vi "Timer2.vi"() -> ()   [LabVIEW 2011]
panel:
  out "String":string
  out "path string":string
  out "read text":string
  in  "save":bool
  out "CurrentPath":path=path "C:/Documents and Settings/TGI0362/My Documents/xUserData/LabVIEW_8.x/cmDVT_Factory-BBU-R5"
  in  "stop":bool
  in  "error in":errorcluster
  out "error out 2":errorcluster
  out "VISA resource name out":refnum<visa-resource-name>
  out "error out":errorcluster
  out "VISA resource 2":refnum<visa-resource-name>
  out "P1.0 status(True=ON)":bool
  out "In Range?":bool
  out "hr+min":i32
  out "OFF hr+min":i32
  out "ON hr+min":i32
  out "Today? \n(True=Enable)":bool
  out "week string":string
  out "now week string":string
  out "confilct ? (True=no conflict)":bool
  in  "OFF minute(00-59)":i32
  in  "OFF hour(00-23)":i32
  in  "ON minute(00-59)":i32
  in  "ON hour(00-23)":i32
  in  "Sun":bool
  in  "Sat":bool
  in  "Fri":bool
  in  "Thu":bool
  in  "Wed":bool
  in  "Tue":bool
  in  "Mon":bool
  out "new picture":picture
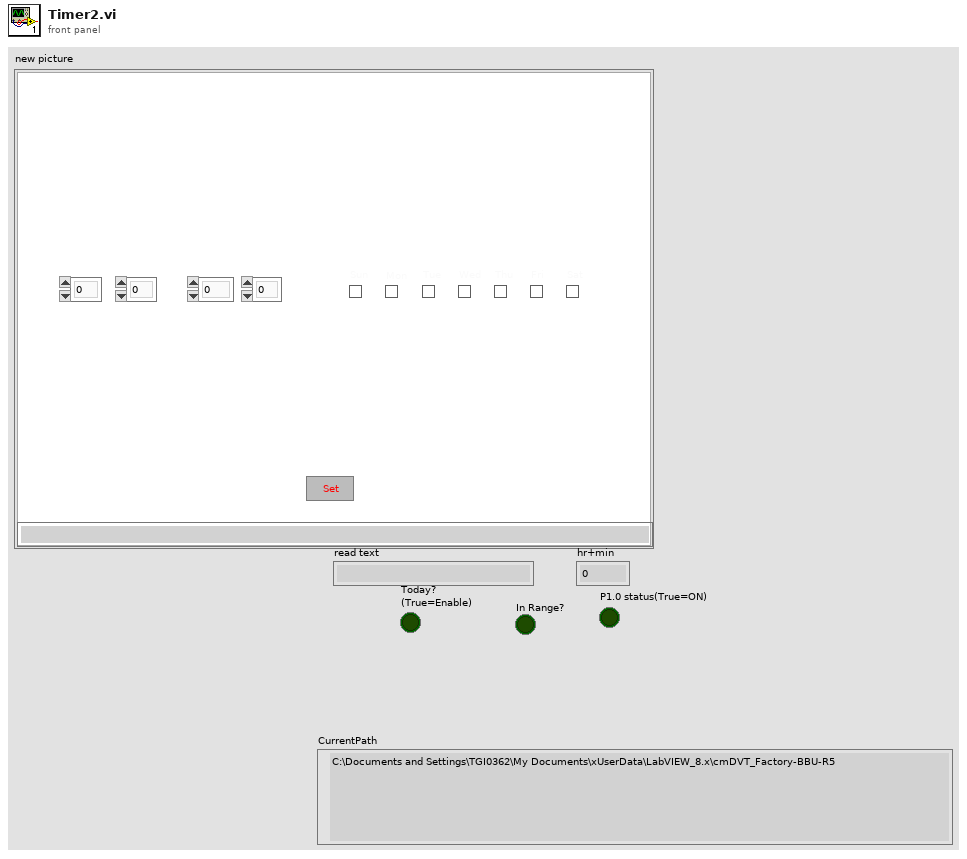
[diagram p1: front panel]
types:
  T1 = typedef "imagedata.ctl" = cluster{"image type":i32, "image depth":i32, "image":u8[], "mask":u8[], "colors":u32[], "Rectangle":cluster{"left":i16, "top":i16, "right":i16, "bottom":i16}}
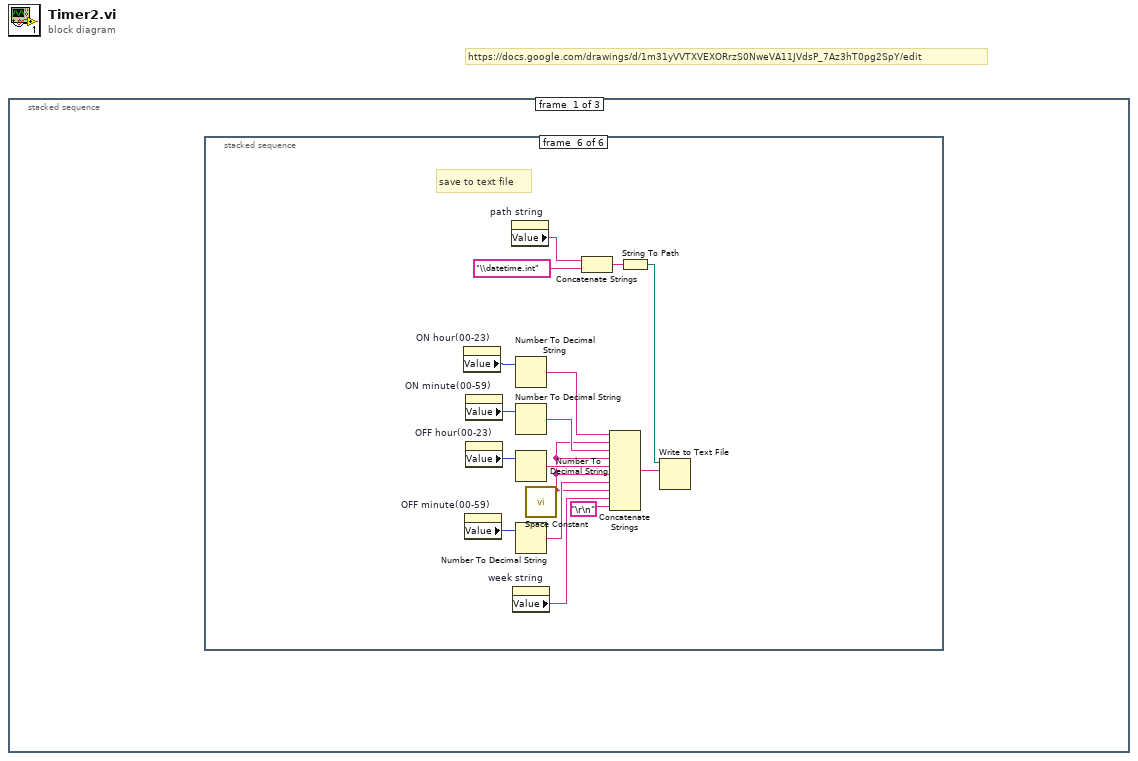
[diagram p0: block diagram]
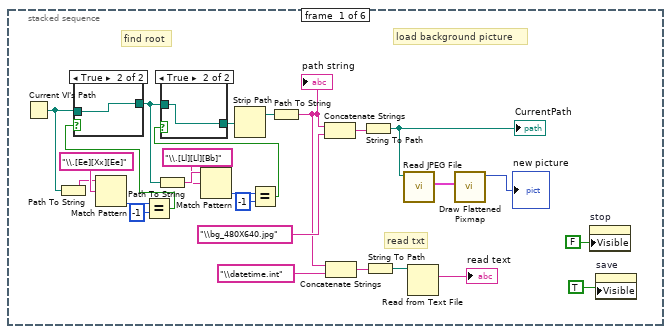
[diagram p2: hidden frame]
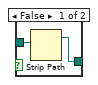
[diagram p3: hidden frame]
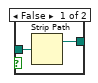
[diagram p4: hidden frame]
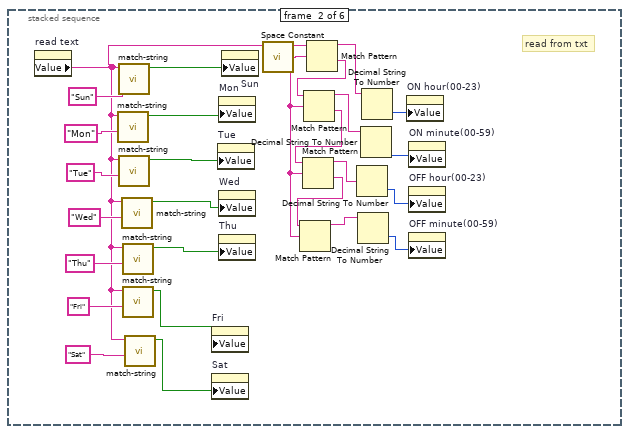
[diagram p5: hidden frame]
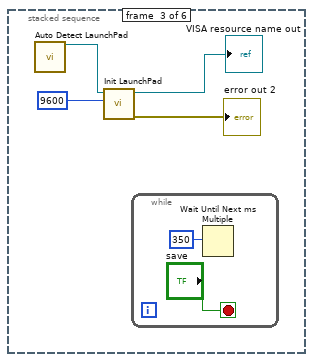
[diagram p6: hidden frame]
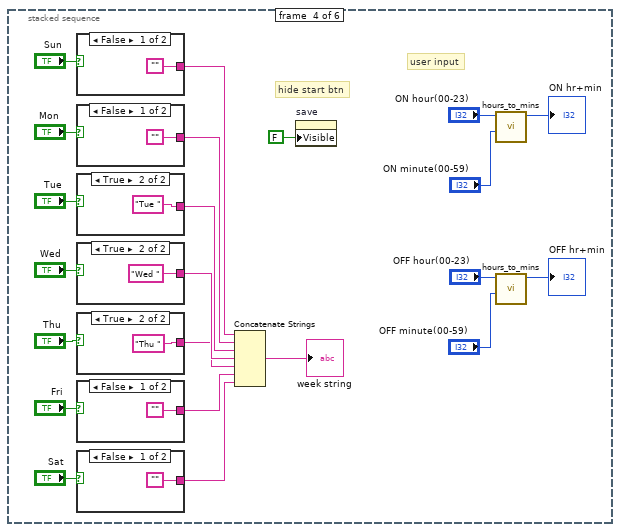
[diagram p7: hidden frame]
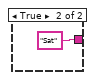
[diagram p8: hidden frame]
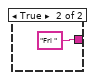
[diagram p9: hidden frame]
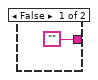
[diagram p10: hidden frame]
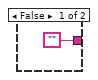
[diagram p11: hidden frame]
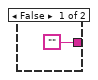
[diagram p12: hidden frame]
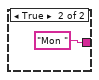
[diagram p13: hidden frame]
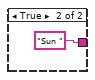
[diagram p14: hidden frame]
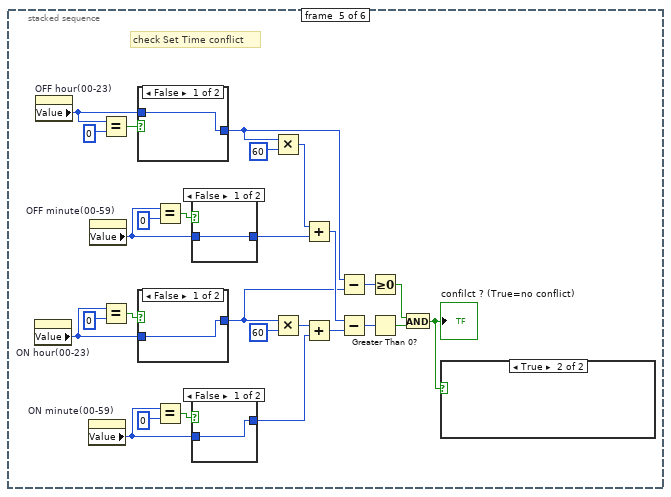
[diagram p15: hidden frame]
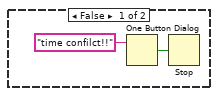
[diagram p16: hidden frame]
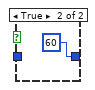
[diagram p17: hidden frame]
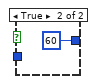
[diagram p18: hidden frame]
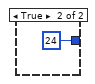
[diagram p19: hidden frame]
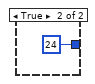
[diagram p20: hidden frame]
diagram:
  # "https://docs.google.com/drawings/d/1m31yVVTXVEXORrzS0NweVA11JVdsP_7Az3hT0pg2SpY/edit"
  n1 = stacked-sequence {
    frame #0 {
      n2 = stacked-sequence {
        frame #0 {
          # "read txt"
          # "load background picture"
          # "find root"
          n3 = Current VI's Path() -> (path=w15:path)
          n4 = Path To String(path=w15) -> (string=w14:string)
          n5 = Match Pattern(string=w14, regular expression="\\.[Ee][Xx][Ee]") -> (offset past match=w12:i32)  [unwired: 1 in, 3 out]
          n6 = Equal?(x=w12, y=-1) -> (x = y?=w24:bool)
          n7 = case shown="True" w24 {
            tunnel: [w30 w32] -> w21
            tunnel: w15 -> [w31 w32]
            frame False {
              n8 = Strip Path(path=w31) -> (stripped path=w30:path)  [unwired: 1 out]
            }
            frame True {
            }
          }
          n9 = Path To String(path=w21) -> (string=w18:string)
          n10 = Match Pattern(string=w18, regular expression="\\.[Ll][Ll][Bb]") -> (offset past match=w20:i32)  [unwired: 1 in, 3 out]
          n11 = Equal?(x=w20, y=-1) -> (x = y?=w23:bool)
          n12 = case shown="True" w23 {
            tunnel: [w27 w29] -> w22
            tunnel: w21 -> [w28 w29]
            frame False {
              n13 = Strip Path(path=w28) -> (stripped path=w27:path)  [unwired: 1 out]
            }
            frame True {
            }
          }
          n14 = Strip Path(path=w22) -> (stripped path=w11:path)  [unwired: 1 out]
          n15 = Path To String(path=w11) -> (string=w1:string)
          "path string" <- w1
          n16 = Concatenate Strings(w1, "\\bg_480X640.jpg") -> (w9:string)
          n17 = Concatenate Strings(w1, "\\datetime.int") -> (w4:string)
          n18 = String To Path(string=w9) -> (path=w8:path)
          "CurrentPath" <- w8
          n19 = String To Path(string=w4) -> (path=w3:path)
          n20 = call <vilib>:"Read JPEG File.vi"("path to JPEG file"=w8) -> ("image data"=w25:T1)  [unwired: 8 in, 2 out]
          n21 = Read from Text File(file (use dialog)=w3) -> (text=→"read text":string)  [unwired: 3 in, 3 out]
          n22 = call <vilib>:"Draw Flattened Pixmap.vi"("image data"=w25) -> ("new picture"=→"new picture":picture)  [unwired: 8 in]
          n23 = property on="stop" class="Bool"("Visible"=FALSE) -> ()  [unwired: 2 in, 2 out]
          n24 = property on="save" class="Bool"("Visible"=TRUE) -> ()  [unwired: 2 in, 2 out]
        }
        frame #1 {
          # "read from txt"
          n25 = property on="read text" class="Str"() -> ("Value"=w45:string)  [unwired: 2 in, 2 out]
          n26 = call "match-string.vi"("match string"="Mon", "String"=w45) -> ("match?(True=match)"=w46:bool)  [unwired: 9 in]
          n27 = call "match-string.vi"("match string"="Sun", "String"=w45) -> ("match?(True=match)"=w59:bool)  [unwired: 9 in]
          n28 = call "match-string.vi"("match string"="Tue", "String"=w45) -> ("match?(True=match)"=w47:bool)  [unwired: 9 in]
          n29 = call "match-string.vi"("match string"="Wed", "String"=w45) -> ("match?(True=match)"=w48:bool)  [unwired: 9 in]
          n30 = call "match-string.vi"("match string"="Thu", "String"=w45) -> ("match?(True=match)"=w49:bool)  [unwired: 9 in]
          n31 = call "match-string.vi"("match string"="Fri", "String"=w45) -> ("match?(True=match)"=w50:bool)  [unwired: 9 in]
          n32 = call "match-string.vi"("match string"="Sat", "String"=w45) -> ("match?(True=match)"=w51:bool)  [unwired: 9 in]
          n33 = property on="Fri" class="Bool (strict)"("Value"=w50) -> ()  [unwired: 2 in, 2 out]
          n34 = property on="Sat" class="Bool (strict)"("Value"=w51) -> ()  [unwired: 2 in, 2 out]
          n35 = property on="Tue" class="Bool (strict)"("Value"=w47) -> ()  [unwired: 2 in, 2 out]
          n36 = property on="Mon" class="Bool (strict)"("Value"=w46) -> ()  [unwired: 2 in, 2 out]
          n37 = property on="Wed" class="Bool (strict)"("Value"=w48) -> ()  [unwired: 2 in, 2 out]
          n38 = property on="Thu" class="Bool (strict)"("Value"=w49) -> ()  [unwired: 2 in, 2 out]
          n39 = property on="Sun" class="Bool (strict)"("Value"=w59) -> ()  [unwired: 2 in, 2 out]
          n40 = call <vilib>:"Space Constant.vi"() -> ("String"=w34:string)
          n41 = Match Pattern(string=w45, regular expression=w34) -> (before substring=w44:string, after substring=w42:string)  [unwired: 1 in, 2 out]
          n42 = Match Pattern(string=w42, regular expression=w34) -> (before substring=w41:string, after substring=w40:string)  [unwired: 1 in, 2 out]
          n43 = Match Pattern(string=w40, regular expression=w34) -> (before substring=w39:string, after substring=w36:string)  [unwired: 1 in, 2 out]
          n44 = Match Pattern(string=w36, regular expression=w34) -> (before substring=w35:string)  [unwired: 1 in, 3 out]
          n45 = Decimal String To Number(string=w39) -> (number=w38:i32)  [unwired: 2 in, 1 out]
          n46 = Decimal String To Number(string=w35) -> (number=w33:i32)  [unwired: 2 in, 1 out]
          n47 = Decimal String To Number(string=w41) -> (number=w37:i32)  [unwired: 2 in, 1 out]
          n48 = Decimal String To Number(string=w44) -> (number=w43:i32)  [unwired: 2 in, 1 out]
          n49 = property on="ON hour(00-23)" class="DigNum (strict)"("Value"=w43) -> ()  [unwired: 2 in, 2 out]
          n50 = property on="ON minute(00-59)" class="DigNum (strict)"("Value"=w37) -> ()  [unwired: 2 in, 2 out]
          n51 = property on="OFF hour(00-23)" class="DigNum (strict)"("Value"=w38) -> ()  [unwired: 2 in, 2 out]
          n52 = property on="OFF minute(00-59)" class="DigNum (strict)"("Value"=w33) -> ()  [unwired: 2 in, 2 out]
        }
        frame #2 {
          n53 = call "Auto Detect LaunchPad.vi"() -> ("VISA resource"=w62:refnum<visa-resource-name>)  [unwired: 14 in, 1 out]
          n54 = call "Init LaunchPad.vi"("Baud Rate (9600)"=u32 9600, "VISA resource"=w62) -> ("error out"=→"error out 2":errorcluster, "VISA resource name out"=→"VISA resource name out":refnum<visa-resource-name>)  [unwired: 8 in]
          n55 = while {
            stop <- "save" stop-if-true
            n56 = Wait Until Next ms Multiple(millisecond multiple=u32 350) -> ()  [unwired: 1 out]
          }
        }
        frame #3 {
          # "hide start btn"
          # "user input"
          n57 = case shown="False" "Sun" {
            tunnel: ["" "Sun "] -> w86
            frame False {
            }
            frame True {
            }
          }
          n58 = case shown="False" "Mon" {
            tunnel: ["" "Mon "] -> w79
            frame False {
            }
            frame True {
            }
          }
          n59 = case shown="True" "Tue" {
            tunnel: ["" "Tue "] -> w78
            frame False {
            }
            frame True {
            }
          }
          n60 = case shown="True" "Wed" {
            tunnel: ["" "Wed "] -> w77
            frame False {
            }
            frame True {
            }
          }
          n61 = case shown="True" "Thu" {
            tunnel: ["" "Thu "] -> w76
            frame False {
            }
            frame True {
            }
          }
          n62 = case shown="False" "Fri" {
            tunnel: ["" "Fri "] -> w75
            frame False {
            }
            frame True {
            }
          }
          n63 = case shown="False" "Sat" {
            tunnel: ["" "Sat"] -> w74
            frame False {
            }
            frame True {
            }
          }
          n64 = Concatenate Strings(w86, w79, w78, w77, w76, w75, w74) -> (→"week string":string)
          n65 = property on="save" class="Bool"("Visible"=FALSE) -> ()  [unwired: 2 in, 2 out]
          n66 = call "hours_to_mins.vi"("minute(00-59)"="ON minute(00-59)", "hour(00-23)"="ON hour(00-23)") -> ("hr+min"=→"ON hr+min":i32)  [unwired: 9 in]
          n67 = call "hours_to_mins.vi"("minute(00-59)"="OFF minute(00-59)", "hour(00-23)"="OFF hour(00-23)") -> ("hr+min"=→"OFF hr+min":i32)  [unwired: 9 in]
        }
        frame #4 {
          # "check Set Time conflict"
          n68 = property on="ON hour(00-23)" class="DigNum (strict)"() -> ("Value"=w121:i32)  [unwired: 2 in, 2 out]
          n69 = property on="OFF hour(00-23)" class="DigNum (strict)"() -> ("Value"=w124:i32)  [unwired: 2 in, 2 out]
          n70 = property on="ON minute(00-59)" class="DigNum (strict)"() -> ("Value"=w118:i32)  [unwired: 2 in, 2 out]
          n71 = property on="OFF minute(00-59)" class="DigNum (strict)"() -> ("Value"=w115:i32)  [unwired: 2 in, 2 out]
          n72 = Equal?(x=w124, y=0) -> (x = y?=w126:bool)
          n73 = Equal?(x=w121, y=0) -> (x = y?=w123:bool)
          n74 = case shown="False" w126 {
            tunnel: [w137 24] -> w111
            tunnel: w124 -> [w137 _]
            frame False {
            }
            frame True {
            }
          }
          n75 = case shown="False" w123 {
            tunnel: [w135 24] -> w105
            tunnel: w121 -> [w135 _]
            frame False {
            }
            frame True {
            }
          }
          n76 = Equal?(x=w115, y=0) -> (x = y?=w117:bool)
          n77 = Equal?(x=w118, y=0) -> (x = y?=w120:bool)
          n78 = case shown="False" w117 {
            tunnel: [w131 60] -> w108
            tunnel: w115 -> [w131 _]
            frame False {
            }
            frame True {
            }
          }
          n79 = case shown="False" w120 {
            tunnel: [w133 60] -> w103
            tunnel: w118 -> [w133 _]
            frame False {
            }
            frame True {
            }
          }
          n80 = Multiply(x=w111, y=60) -> (x*y=w109:i32)
          n81 = Multiply(x=w105, y=60) -> (x*y=w104:i32)
          n82 = Add(x=w109, y=w108) -> (x+y=w107:i32)
          n83 = Add(x=w104, y=w103) -> (x+y=w102:i32)
          n84 = Subtract(x=w111, y=w105) -> (x-y=w128:i32)
          n85 = Subtract(x=w107, y=w102) -> (x-y=w127:i32)
          n86 = Greater Or Equal To 0?(x=w128) -> (x >= 0?=w114:bool)
          n87 = Greater Than 0?(x=w127) -> (x > 0?=w113:bool)
          n88 = And(x=w114, y=w113) -> (x .and. y?=w112:bool)
          "confilct ? (True=no conflict)" <- w112
          n89 = case shown="True" w112 {
            frame False {
              n90 = One Button Dialog(message="time confilct!!") -> (true=w129:bool)  [unwired: 1 in]
              n91 = Stop(stop? (T)=w129) -> ()
            }
            frame True {
            }
          }
        }
        frame #5 {
          # "save to text file"
          n92 = property on="ON hour(00-23)" class="DigNum (strict)"() -> ("Value"=w142:i32)  [unwired: 2 in, 2 out]
          n93 = property on="OFF minute(00-59)" class="DigNum (strict)"() -> ("Value"=w139:i32)  [unwired: 2 in, 2 out]
          n94 = property on="ON minute(00-59)" class="DigNum (strict)"() -> ("Value"=w141:i32)  [unwired: 2 in, 2 out]
          n95 = property on="OFF hour(00-23)" class="DigNum (strict)"() -> ("Value"=w140:i32)  [unwired: 2 in, 2 out]
          n96 = property on="path string" class="Str"() -> ("Value"=w144:string)  [unwired: 2 in, 2 out]
          n97 = property on="week string" class="Str"() -> ("Value"=w150:string)  [unwired: 2 in, 2 out]
          n98 = Number To Decimal String(number=w142) -> (decimal integer string=w154:string)  [unwired: 1 in]
          n99 = Number To Decimal String(number=w141) -> (decimal integer string=w153:string)  [unwired: 1 in]
          n100 = Number To Decimal String(number=w140) -> (decimal integer string=w152:string)  [unwired: 1 in]
          n101 = Number To Decimal String(number=w139) -> (decimal integer string=w151:string)  [unwired: 1 in]
          n102 = call <vilib>:"Space Constant.vi"() -> ("String"=w149:string)
          n103 = Concatenate Strings(w144, "\\datetime.int") -> (w145:string)
          n104 = Concatenate Strings(w154, w149, w153, w149, w152, w149, w151, w149, w150, "\r\n") -> (w148:string)
          n105 = String To Path(string=w145) -> (path=w143:path)
          n106 = Write to Text File(file (use dialog)=w143, text=w148) -> ()  [unwired: 2 in, 3 out]
        }
      }
    }
    frame #1 {
      n107 = while {
        stop <- "stop" stop-if-true
        n108 = stacked-sequence {
          frame #0 {
            # "Is time in range?"
            # "Is  today?"
            n109 = property on="stop" class="Bool"("Visible"=TRUE) -> ()  [unwired: 2 in, 2 out]
            n110 = Get Date/Time In Seconds "current Time"() -> (seconds since 1Jan1904=w161:timestamp)
            n111 = property on="week string" class="Str"() -> ("Value"=w167:string)  [unwired: 2 in, 2 out]
            n112 = Format Date/Time String(time format string (%c)="%a", seconds (now)=w161) -> (date/time string=w166:string)  [unwired: 1 in]
            "now week string" <- w166
            n113 = Match Pattern(string=w167, regular expression=w166) -> (match substring=w165:string)  [unwired: 1 in, 3 out]
            n114 = String Length(string=w165) -> (length=w164:i32)
            n115 = Not Equal To 0?(x=w164) -> (x != 0?=w162:bool)
            "Today? \n(True=Enable)" <- w162
            n116 = case shown="True" w162 {
              selector: w162 -> [w170 _]
              tunnel: [w170 w172] -> w169
              tunnel: w161 -> [_ w171]
              frame False {
              }
              frame True {
                # "Hour+Minute in range?"
                n117 = property on="OFF hr+min" class="DigNum (strict)"() -> ("Value"=w174:i32)  [unwired: 2 in, 2 out]
                n118 = property on="ON hr+min" class="DigNum (strict)"() -> ("Value"=w175:i32)  [unwired: 2 in, 2 out]
                n119 = call "TrimHourMin.vi"("Time"=w171) -> ("hr+min"=w173:i32)  [unwired: 8 in, 2 out]
                "hr+min" <- w173
                n120 = In Range and Coerce(upper limit=w174, x=w173, lower limit=w175) -> (In Range?=w172:bool)  [unwired: 1 out]
              }
            }
            "In Range?" <- w169
          }
          frame #1 {
            # "LabVIEW Interface for LaunchPad (LILP_MSP430G2553) v1\n#define            M_D0        0x30   // Char ASCII \"0\"\n#define            M_A4        0x34   // Char ASCII \"4\""
            # "1000"
            # "check P1.0 status by P1.4 analog (if ON P1.4=1000, if OFF=0000)"
            n121 = property on="error out 2" class="Clust (strict)"() -> ("Value"=w177:errorcluster)  [unwired: 2 in, 2 out]
            n122 = property on="VISA resource name out" class="VISAName"() -> ("Value"=w178:refnum<visa-resource-name>)  [unwired: 2 in, 2 out]
            n123 = call "Send Receive LaunchPad.vi"("VISA resource"=w178, "write buffer"="4", "Bytes To Read (0)"=u8 2, "Max Retries  (10)"=1, "error in"=w177) -> ("VISA resource 2"=→"VISA resource 2":refnum<visa-resource-name>, "Read Buffer"=w184:string, "error out"=→"error out":errorcluster)  [unwired: 8 in]
            n124 = call "ADC10 LaunchPad.vi"("string"=w184) -> ("ADCvalue"=w182:u16)  [unwired: 9 in, 1 out]
            n125 = Greater?(x=w182, y=u16 900) -> (0:w176:bool)
            "P1.0 status(True=ON)" <- w176
            n126 = case shown="False" w176 {
              frame False {
                n127 = property on="In Range?" class="Bool (strict)"() -> ("Value"=w187:bool)  [unwired: 2 in, 2 out]
                n128 = case shown="True" w187 {
                  frame False {
                    # "do nothing"
                  }
                  frame True {
                    # "need toggle to turn ON"
                    n129 = property on="VISA resource 2" class="VISAName"() -> ("Value"=w190:refnum<visa-resource-name>)  [unwired: 2 in, 2 out]
                    n130 = property on="error out" class="Clust (strict)"() -> ("Value"=w189:errorcluster)  [unwired: 2 in, 2 out]
                    n131 = call "Send Receive LaunchPad.vi"("VISA resource"=w190, "write buffer"="0", "Bytes To Read (0)"=u8 2, "Max Retries  (10)"=1, "error in"=w189) -> ("error out"=w188:errorcluster)  [unwired: 8 in, 2 out]
                    n132 = property on="error in" class="Clust (strict)"("Value"=w188) -> ()  [unwired: 2 in, 2 out]
                  }
                }
              }
              frame True {
                n133 = property on="In Range?" class="Bool (strict)"() -> ("Value"=w194:bool)  [unwired: 2 in, 2 out]
                n134 = case shown="False" w194 {
                  frame False {
                    # "in error action , try to toggle trun off"
                    n135 = property on="VISA resource 2" class="VISAName"() -> ("Value"=w197:refnum<visa-resource-name>)  [unwired: 2 in, 2 out]
                    n136 = property on="error out" class="Clust (strict)"() -> ("Value"=w196:errorcluster)  [unwired: 2 in, 2 out]
                    n137 = call "Send Receive LaunchPad.vi"("VISA resource"=w197, "write buffer"="0", "Bytes To Read (0)"=u8 2, "Max Retries  (10)"=1, "error in"=w196) -> ("error out"=w195:errorcluster)  [unwired: 8 in, 2 out]
                    n138 = property on="error in" class="Clust (strict)"("Value"=w195) -> ()  [unwired: 2 in, 2 out]
                  }
                  frame True {
                    # "do nothing"
                  }
                }
              }
            }
          }
        }
        n139 = Format Date/Time String(time format string (%c)="%Y - %m - %d   %H : %M : %S") -> (date/time string=w157:string)  [unwired: 2 in]
        n140 = Wait Until Next ms Multiple(millisecond multiple=u32 1000) -> ()  [unwired: 1 out]
        n141 = Concatenate Strings("現在時間:   ", w157) -> (→"String":string)
      }
    }
    frame #2 {
      n142 = property on="VISA resource name out" class="VISAName"() -> ("Value"=w202:refnum<visa-resource-name>)  [unwired: 2 in, 2 out]
      n143 = call "Close LaunchPad.vi"("VISA resource name"=w202, "error in"="error in") -> ()  [unwired: 13 in, 1 out]
      n144 = property on="save" class="Bool"("Visible"=TRUE) -> ()  [unwired: 2 in, 2 out]
    }
  }
